vi "DSF.Engine.Transceiver Thread.Get Channels Buffer.vi"(11 "Transceiver Thread in":refnum<class "DSF.Engine.Transceiver Thread.lvclass">) -> (2 "channels buffer":dbl[](array[numeric]), 3 "Transceiver Thread out":refnum<class "DSF.Engine.Transceiver Thread.lvclass">)   [LabVIEW 2017, in "Data Sharing Framework Engine.lvlib" / "DSF.Engine.Transceiver Thread.lvclass"]
uses:
  DSF.Engine.Transceiver Thread.lvclass
  DSF.Engine.Transceiver Thread.lvclass/DSF.Engine.Transceiver Thread.ctl
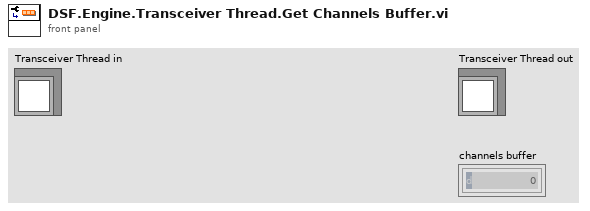
[diagram p1: front panel]
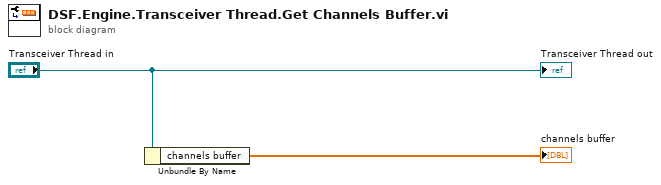
[diagram p0: block diagram]
diagram:
  n1 = Unbundle By Name("Transceiver Thread in") -> ("channels buffer"=→"channels buffer":dbl[])
  "Transceiver Thread out" <- "Transceiver Thread in"
